vi "Get_No_Top_Level_Message.vi"(11 "Build in":refnum<class "AB_EXE.lvclass">) -> (2 "No top level VI":string, 3 "Build out":refnum<class "AB_EXE.lvclass">)   [LabVIEW 2020, in "AB_EXE.lvclass"]
uses:
  <vilib>/AppBuilder/AB_Classes/EXE/AB_EXE.lvclass
  <vilib>/AppBuilder/AB_Classes/EXE/AB_EXE.lvclass/AB_EXE.ctl
  <resource>/Framework/Providers/Common/provcom_StringGlobals.vi
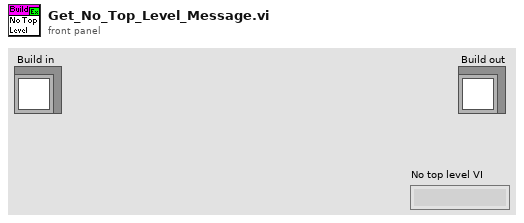
[diagram p1: front panel]
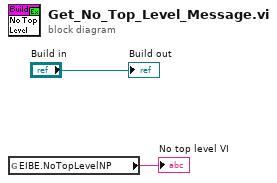
[diagram p0: block diagram]
diagram:
  n1 = global read "provcom_StringGlobals.vi" "EIBE.NoTopLevelNP"() -> (→"No top level VI":string)
  "Build out" <- "Build in"
